vi "sin_A_cos_a.vi"(1 "AH":dbl, 2 "DEC":dbl) -> (0 "sinAcosa":dbl)   [LabVIEW 2012]
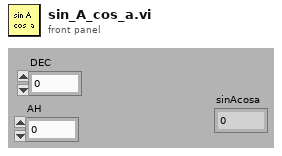
[diagram p1: front panel]
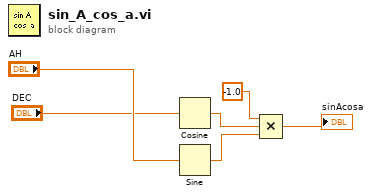
[diagram p0: block diagram]
diagram:
  n1 = Cosine(x="DEC") -> (cos(x)=w4:dbl)
  n2 = Sine(x="AH") -> (sin(x)=w5:dbl)
  n3 = Compound Arithmetic op=MULTIPLY(-1.0 ("value"), w4, w5) -> (→"sinAcosa":dbl)
